vi "ToshibaComms.vi"(0 "FPGA VI Reference In":T8, 1 "PC Data In":T7, 3 "ES String Data Array In":T3, 4 "ES System Data In":T5={"Voltage"=0.0, "Current"=0.0, "SOC Avg"=0.0, "Faults"=0, "Alarms"=0, "Number of Strings"=0, "Max Temp"=0, "Min Temp"=0, "Max Cell Voltage"=0.0, "Min Cell Voltage"=0.0, "Energy Capacity (kWh)"=0.0, "Energy Remaining (kWh)"=0.0, "SOC Min"=0.0, "SOC Max"=0.0, "ES Fault"=FALSE, "String Selector"=enum."3 Strings"}, 5 "Error In":errorcluster, 6 "Contactor 2 Closed?":bool, 8 "Contactor 1 Closed?":bool) -> (10 "String A Com Fault":bool, 11 "Module Indicators 1":T1, 12 "String B Com Fault":bool, 14 "FPGA VI Reference Out":T8, 15 "Current Limit Parameters Out":T2, 17 "ES String Data Array Out":T3, 18 "ES System Data Out":T5={"Voltage"=0.0, "Current"=0.0, "SOC Avg"=0.0, "Faults"=0, "Alarms"=0, "Number of Strings"=0, "Max Temp"=0, "Min Temp"=0, "Max Cell Voltage"=0.0, "Min Cell Voltage"=0.0, "Energy Capacity (kWh)"=0.0, "Energy Remaining (kWh)"=0.0, "SOC Min"=0.0, "SOC Max"=0.0, "ES Fault"=FALSE, "String Selector"=enum."3 Strings"}, 19 "Error Out":errorcluster)   [LabVIEW 2013]
uses:
  bigboss/trunk/sw/cRIO/Controls/FPGAReference BigBoss.ctl
  eng/trunk/ni/cRIO Master Files/Controls/PowerConversionData.ctl
  eng/trunk/ni/cRIO Master Files/Controls/EnergyStorageSystemData.ctl
  eng/trunk/ni/cRIO Master Files/Controls/StringSelector.ctl
  eng/trunk/ni/cRIO Master Files/Controls/EnergyStorageStringDataArray.ctl
  eng/trunk/ni/cRIO Master Files/Controls/EnergyStorageStringData.ctl
  eng/trunk/ni/cRIO Master Files/Controls/CurrentLimitParameters.ctl
  <vilib>/rvi/interface/nirviMethod/nirviMethod.xnode
  Builds/FPGA Bitfiles/FPGA BIGBOSS.lvbitx
  <vilib>/rvi/errors/niLvFpgaMergeErrorWithErrorCode.vi
  <vilib>/FPGAPlugInAG/cRIO-9068/niLvFpga_ReadFifo_cRIO-9068.vi
  <vilib>/FPGAPlugInAG/cRIO-9068/niLvFpga_WriteFifo_cRIO-9068.vi
panel:
  out "Module Indicators 2":T1
  out "BMU heartbeat 2":bool
  out "BMU heartbeat 1":bool
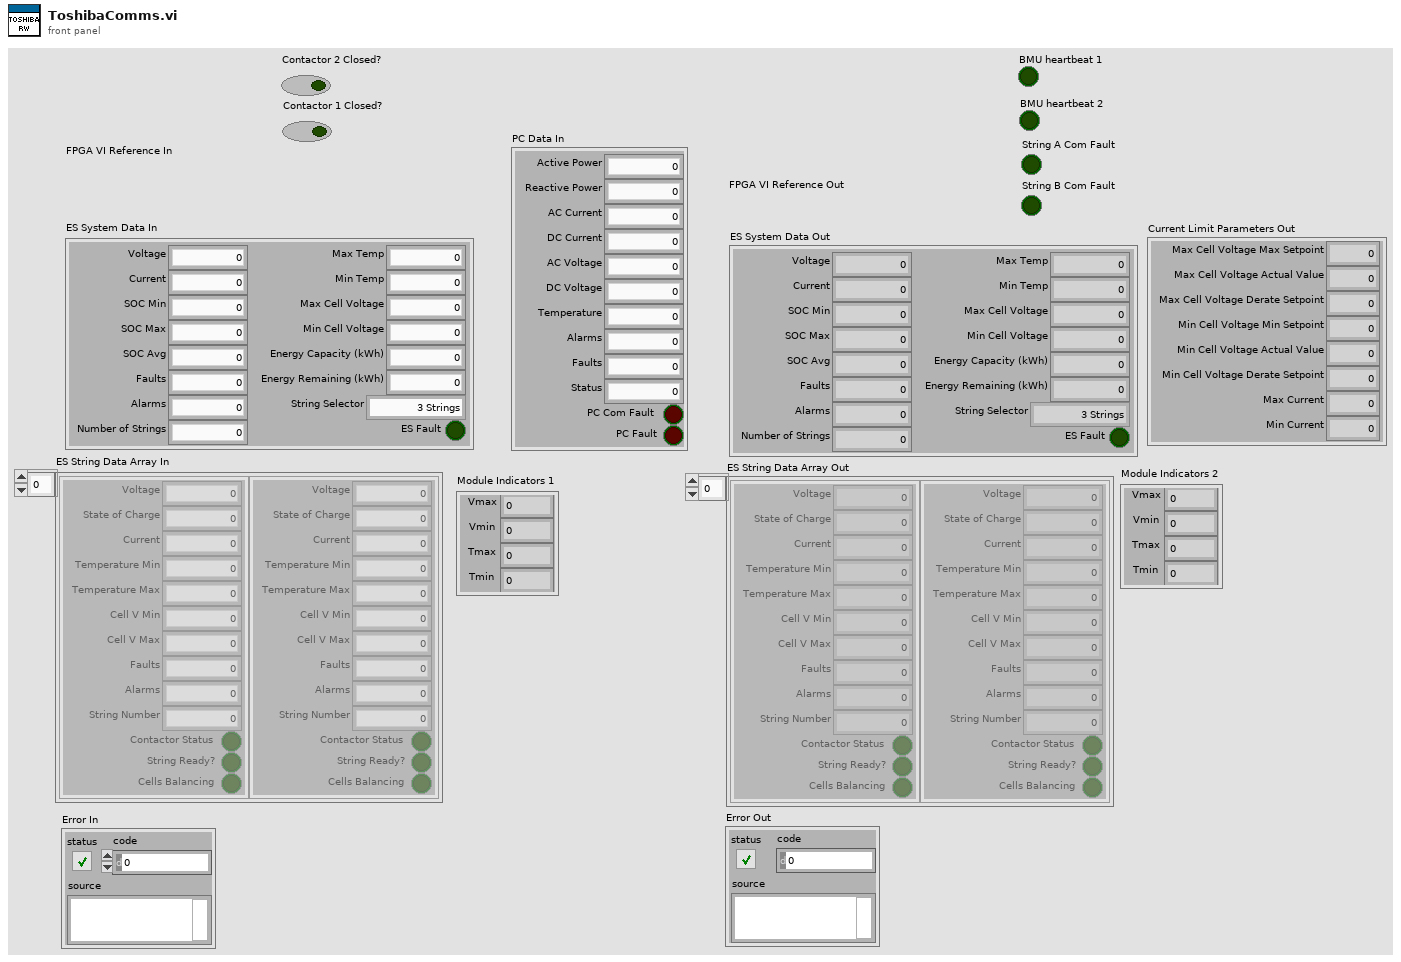
[diagram p1: front panel]
types:
  T1 = cluster{"Vmax":i16, "Vmin":i16, "Tmax":i16, "Tmin":i16}
  T2 = typedef "CurrentLimitParameters.ctl" = cluster{"Max Cell Voltage Max Setpoint":dbl, "Max Cell Voltage Actual Value":dbl, "Max Cell Voltage Derate Setpoint":dbl, "Min Cell Voltage Min Setpoint":dbl, "Min Cell Voltage Actual Value":dbl, "Min Cell Voltage Derate Setpoint":dbl, "Max Current":dbl, "Min Current":dbl}
  T3 = typedef "EnergyStorageStringDataArray.ctl" = T4[]
  T4 = typedef "EnergyStorageStringData.ctl" = cluster{"Voltage":sgl, "State of Charge":sgl, "Current":sgl, "Temperature Min":i16, "Temperature Max":i16, "Faults":u16, "Alarms":u16, "String Number":u16, "Contactor Status":bool, "String Ready?":bool, "Cells Balancing":bool, "Cell V Max":dbl, "Cell V Min":dbl}
  T5 = typedef "EnergyStorageSystemData.ctl" = cluster{"Voltage":sgl, "Current":sgl, "SOC Avg":sgl, "Faults":u16, "Alarms":u16, "Number of Strings":u16, "Max Temp":i16, "Min Temp":i16, "Max Cell Voltage":sgl, "Min Cell Voltage":sgl, "Energy Capacity (kWh)":sgl, "Energy Remaining (kWh)":sgl, "SOC Min":sgl, "SOC Max":sgl, "ES Fault":bool, "String Selector":T6}
  T6 = typedef "StringSelector.ctl" = enum16{"1 String (1)", "1 String (2)", "1 String (3)", "2 Strings (1, 2)", "2 Strings (2, 3)", "2 Strings (1, 3)", "3 Strings"}
  T7 = typedef "PowerConversionData.ctl" = cluster{"Active Power":sgl, "Reactive Power":sgl, "AC Current":sgl, "DC Current":sgl, "AC Voltage":sgl, "DC Voltage":sgl, "Temperature":sgl, "Alarms":u16, "Faults":u16, "Status":u16, "PC Fault":bool, "PC Com Fault":bool}
  T8 = typedef "FPGAReference BigBoss.ctl" = refnum<k20>
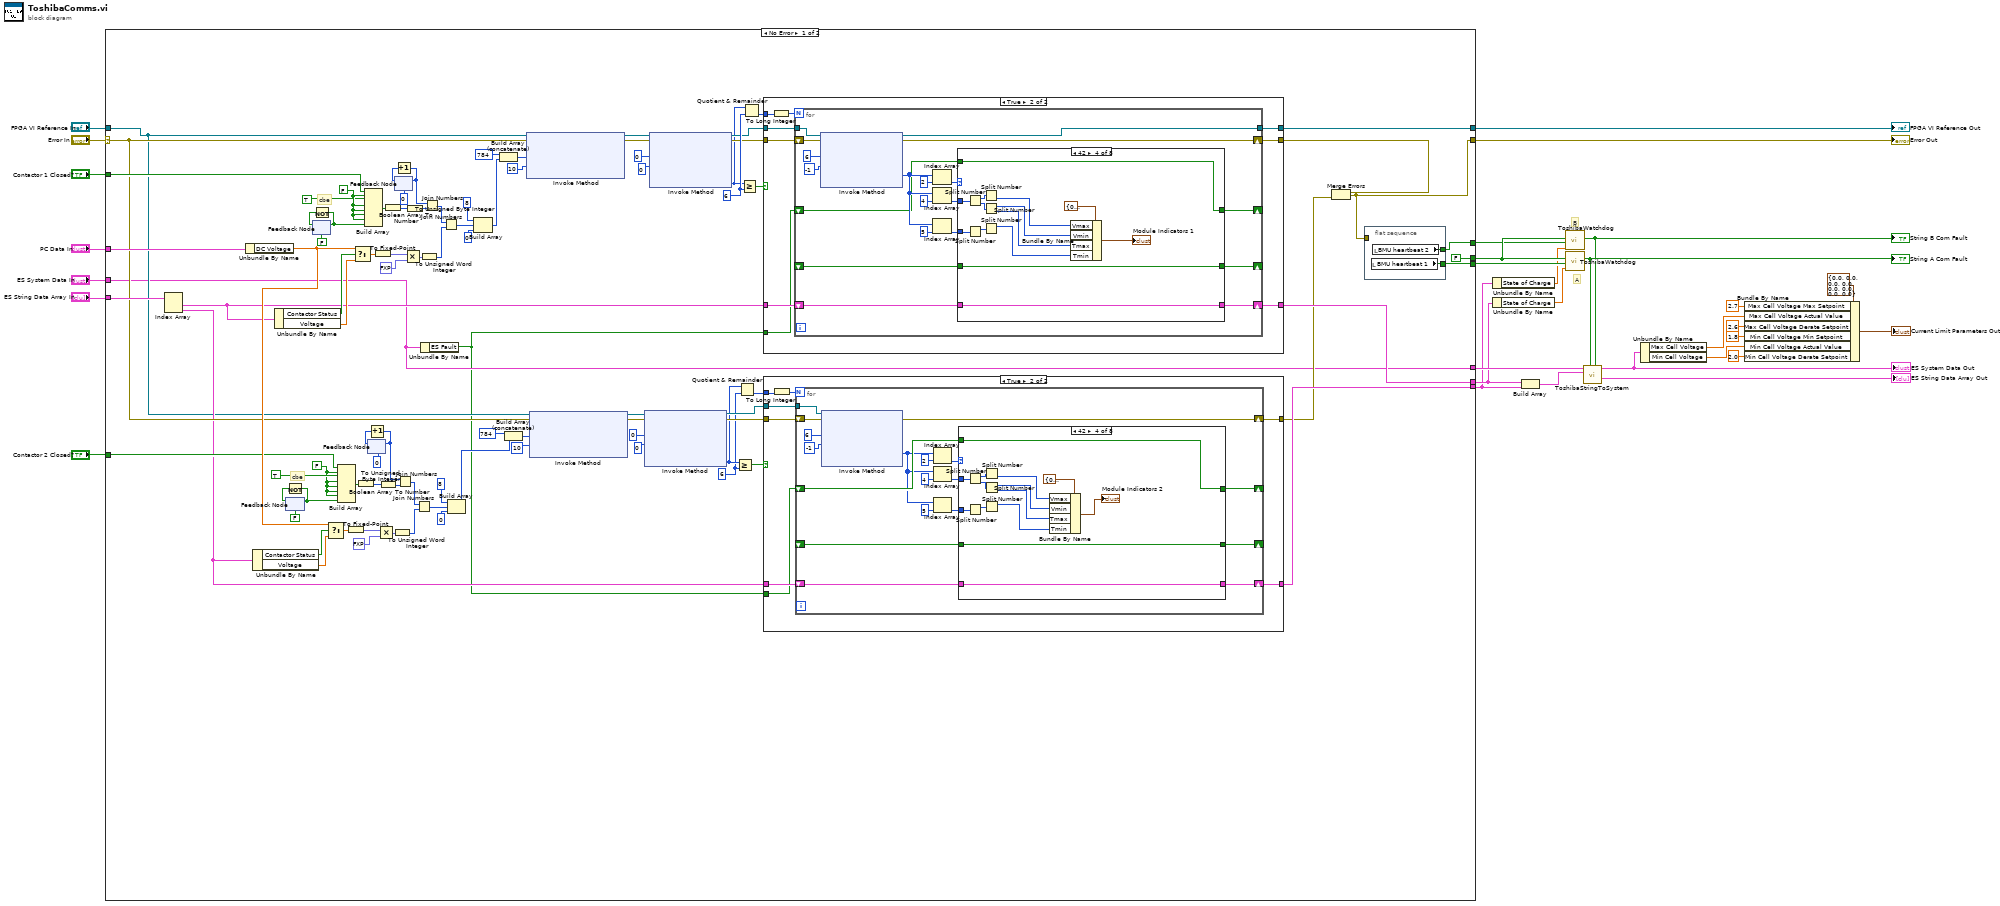
[diagram p0: block diagram]
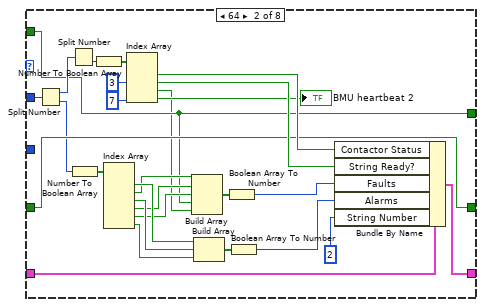
[diagram p4: hidden frame]
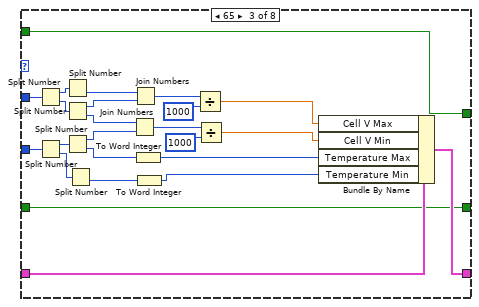
[diagram p5: hidden frame]
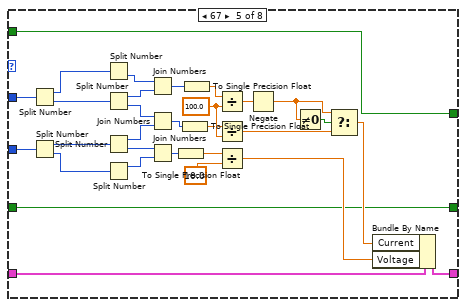
[diagram p6: hidden frame]
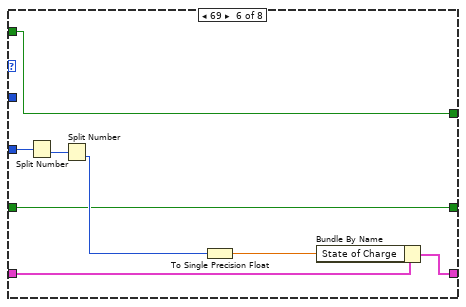
[diagram p7: hidden frame]
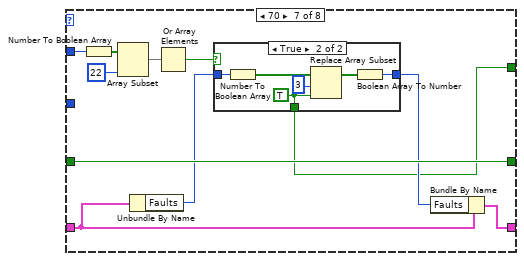
[diagram p8: hidden frame]
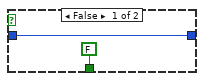
[diagram p9: hidden frame]
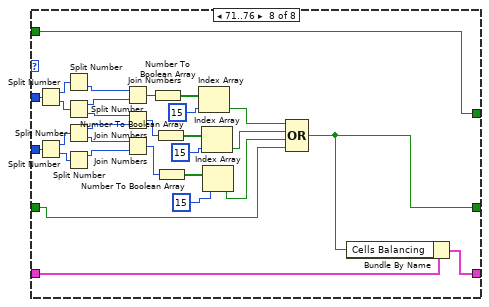
[diagram p10: hidden frame]
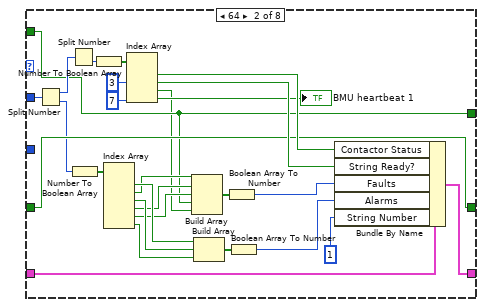
[diagram p13: hidden frame]
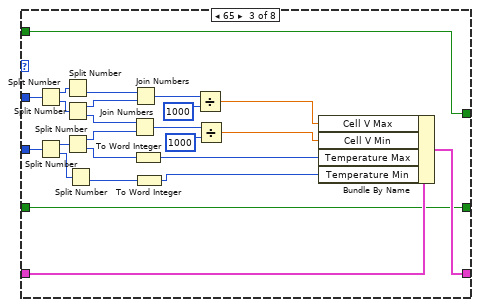
[diagram p14: hidden frame]
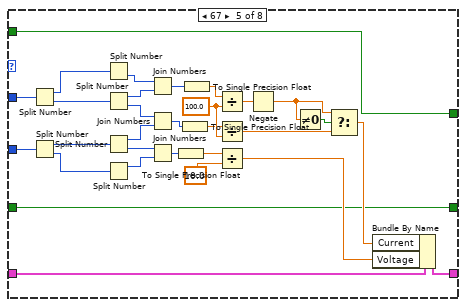
[diagram p15: hidden frame]
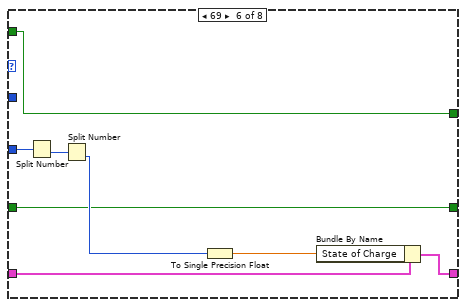
[diagram p16: hidden frame]
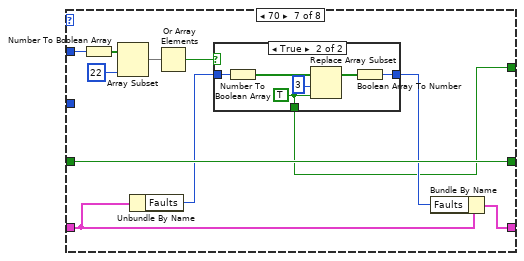
[diagram p17: hidden frame]
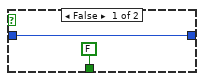
[diagram p18: hidden frame]
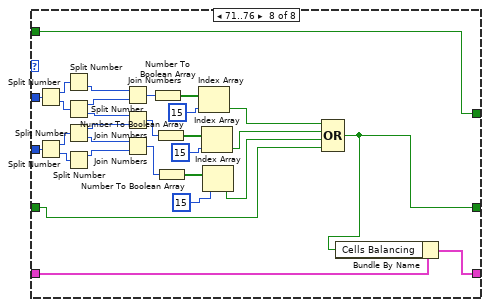
[diagram p19: hidden frame]
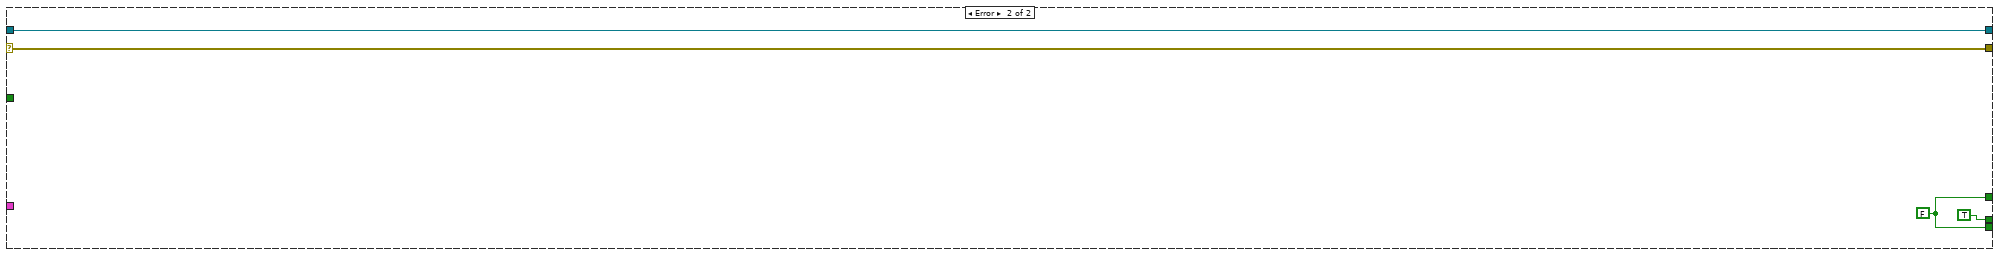
[diagram p20: hidden frame]
diagram:
  # "B"
  # "A"
  n1 = case shown="No Error" "Error In" {
    selector: "Error In" -> [w79 w495]
    tunnel: "FPGA VI Reference In" -> [w33 w494]
    tunnel: [w34 w494] -> w29
    tunnel: [w71 w495] -> w28
    tunnel: "PC Data In" -> [w122 _]
    tunnel: "Contactor 1 Closed?" -> [w121 _]
    tunnel: "ES System Data In" -> [w32 _]
    tunnel: [w32 _] -> w9
    tunnel: [FALSE TRUE] -> w12
    tunnel: "ES String Data Array In" -> [w82 _]
    tunnel: [w119 w492] -> w14
    tunnel: "Contactor 2 Closed?" -> [w86 _]
    tunnel: [w78 w492] -> w11
    tunnel: [w75 _] -> w6
    tunnel: [w74 _] -> w5
    frame No Error {
      w37 = u32 6 ("y")
      w49 = FALSE (".not. x?")
      w106 = FALSE (".not. x?")
      w118 = u32 6 ("y")
      # "cbe"
      # "cbe"
      n2 = Index Array(array=w82) -> (element #1=w77:T4, element #2=w76:T4)  [unwired: 2 in]
      n3 = Unbundle By Name(w122) -> ("DC Voltage"=w87:sgl)
      n4 = Unbundle By Name(w76) -> ("Contactor Status"=w45:bool, "Voltage"=w46:sgl)
      n5 = Unbundle By Name(w77) -> ("Contactor Status"=w84:bool, "Voltage"=w83:sgl)
      n6 = feedback #1(FALSE) -> (w60:bool)
      n7 = Not(x=w60) -> (.not. x?=w59:bool)
      n8 = feedback-in #1(w59) -> ()
      n9 = feedback #2(FALSE) -> (w95:bool)
      n10 = Not(x=w95) -> (.not. x?=w96:bool)
      n11 = feedback-in #2(w96) -> ()
      n12 = Select(t=w87, s=w45, f=w46) -> (s? t:f=w67:sgl)
      n13 = Build Array(w86, w49, TRUE ("Cell Balance 2"), w49, w49, w49, w49, w59) -> (w52:bool[])
      n14 = To Fixed-Point(number=w67) -> (fixed-point=w48:fxp<+,16,9>)  [unwired: 1 in]
      n15 = Select(t=w87, s=w84, f=w83) -> (s? t:f=w88:sgl)
      n16 = Boolean Array To Number(Boolean array=w52) -> (number=w51:u32)
      n17 = Build Array(w121, w106, TRUE, w106, w106, w106, w106, w96) -> (w103:bool[])
      n18 = feedback #3(u8 0) -> (w62:u8)
      n19 = Increment(x=w62) -> (x+1=w63:u8)
      n20 = feedback-in #3(w63) -> ()
      n21 = To Fixed-Point(number=w88) -> (fixed-point=w107:fxp<+,16,9>)  [unwired: 1 in]
      n22 = Multiply(x=w48, y=fxp<+,16,9> 10.0) -> (x*y=w54:fxp<+,16,16>)
      n23 = To Unsigned Byte Integer(number=w51) -> (unsigned 8bit integer=w50:u8)
      n24 = Boolean Array To Number(Boolean array=w103) -> (number=w104:u32)
      n25 = To Unsigned Word Integer(number=w54) -> (unsigned 16bit integer=w53:u16)
      n26 = feedback #4(u8 0) -> (w92:u8)
      n27 = Increment(x=w92) -> (x+1=w91:u8)
      n28 = feedback-in #4(w91) -> ()
      n29 = Join Numbers(hi=w63, lo=w50) -> ((hi.lo)=w56:u16)
      n30 = Multiply(x=w107, y=fxp<+,16,9> 10.0) -> (x*y=w101:fxp<+,16,16>)
      n31 = To Unsigned Byte Integer(number=w104) -> (unsigned 8bit integer=w105:u8)
      n32 = Join Numbers(hi=w56, lo=w53) -> ((hi.lo)=w66:u32)
      n33 = To Unsigned Word Integer(number=w101) -> (unsigned 16bit integer=w102:u16)
      n34 = Unbundle By Name(w32) -> ("ES Fault"=w31:bool)
      n35 = Join Numbers(hi=w91, lo=w105) -> ((hi.lo)=w99:u16)
      n36 = Join Numbers(hi=w99, lo=w102) -> ((hi.lo)=w89:u32)
      n37 = Build Array(u32 8, w66, u32 0 ("CAN Word 2")) -> (w47:u32[])
      n38 = Build Array(u32 8, w89, u32 0 ("CAN Word 2")) -> (w94:u32[])
      n39 = Build Array (concatenate)(u32 784, w94) -> (w109:u32[])
      n40 = Build Array (concatenate)(u32 784, w47) -> (w69:u32[])
      n41 = xnode "Invoke Method"("FPGA VI Reference In"=w33, "error in"=w79, "Data"=w109, "Timeout (ms)"=10) -> ("FPGA VI Reference Out"=w81:T8, "error out"=w80:errorcluster)  [unwired: 1 out]
      n42 = xnode "Invoke Method"("FPGA VI Reference In"=w33, "error in"=w79, "Data"=w69, "Timeout (ms)"=10) -> ("FPGA VI Reference Out"=w42:T8, "error out"=w41:errorcluster)  [unwired: 1 out]
      n43 = xnode "Invoke Method"("FPGA VI Reference In"=w42, "error in"=w41, "Number of Elements"=u32 0, "Timeout (ms)"=0) -> ("FPGA VI Reference Out"=w39:T8, "error out"=w40:errorcluster, "Elements Remaining"=w38:u32)  [unwired: 1 out]
      n44 = xnode "Invoke Method"("FPGA VI Reference In"=w81, "error in"=w80, "Number of Elements"=u32 0, "Timeout (ms)"=0) -> ("FPGA VI Reference Out"=w114:T8, "error out"=w115:errorcluster, "Elements Remaining"=w111:u32)  [unwired: 1 out]
      n45 = Greater Or Equal?(x=w38, y=w37) -> (x >= y?=w35:bool)
      n46 = Quotient & Remainder(x=w38, y=w37) -> (floor(x/y)=w36:u32)  [unwired: 1 out]
      n47 = Greater Or Equal?(x=w111, y=w118) -> (x >= y?=w113:bool)
      n48 = Quotient & Remainder(x=w111, y=w118) -> (floor(x/y)=w112:u32)  [unwired: 1 out]
      n49 = case shown="True" w113 {
        tunnel: w115 -> [w308 w318]
        tunnel: w114 -> [w309 w317]
        tunnel: w112 -> [_ w316]
        tunnel: [w308 w314] -> w72
        tunnel: [w309 w313] -> w34
        tunnel: [w307 w311] -> w75
        tunnel: w77 -> [w307 w312]
        tunnel: w31 -> [_ w310]
        frame False {
        }
        frame True {
          n50 = To Long Integer(number=w316) -> (32bit integer=w315:i32)
          n51 = for {
            N: w315 -> [_]
            tunnel: w317 -> [w337]
            tunnel: [w334] -> w313
            shift-right: [w332] -> w314
            shift-left: w318 -> [w333]
            shift-right: [w320] -> w311
            shift-left: w312 -> [w321]
            shift-right: [w325] -> _
            shift-left: _ -> [w324]
            shift-right: [w323] -> _
            shift-left: w310 -> [w322]
            n52 = xnode "Invoke Method"("FPGA VI Reference In"=w337, "error in"=w333, "Number of Elements"=u32 6, "Timeout (ms)"=-1) -> ("FPGA VI Reference Out"=w334:T8, "error out"=w332:errorcluster, "Data"=w326:u32[])  [unwired: 1 out]
            n53 = Index Array(array=w326, index=2) -> (element=w319:u32)
            n54 = Index Array(array=w326, index=4) -> (element=w330:u32)
            n55 = Index Array(array=w326, index=5) -> (element=w331:u32)
            n56 = case shown="42" w319 {
              tunnel: w330 -> [_ w364 w391 w405 w435 _ w450 w491]
              tunnel: w331 -> [_ _ w387 w401 w431 w443 _ w490]
              tunnel: w321 -> [w340 w357 w377 w398 w415 w439 w444 w467]
              tunnel: [w340 w358 w376 w398 w414 w438 w449 w466] -> w320
              tunnel: [w339 w356 w375 w399 w413 w437 w454 w464] -> w325
              tunnel: w324 -> [w339 w356 w375 w399 w413 w437 w454 w465]
              tunnel: [w338 w342 w370 w400 w406 w436 w445 w463] -> w323
              tunnel: w322 -> [w338 w342 w370 w400 w406 w436 _ w463]
              frame 0, Default {
              }
              frame 64 {
                n57 = Split Number(x=w364) -> (hi(x)=w366:u16, lo(x)=w354:u16)
                n58 = Split Number(x=w366) -> (lo(x)=w365:u8)  [unwired: 1 out]
                n59 = Number To Boolean Array(number=w354) -> (Boolean array=w353:bool[])
                n60 = Number To Boolean Array(number=w365) -> (Boolean array=w367:bool[])
                n61 = Index Array(array=w353) -> (element #1=w352:bool, element #2=w348:bool, element #3=w351:bool, element #4=w347:bool, element #5=w346:bool, element #6=w350:bool)  [unwired: 6 in]
                n62 = Index Array(array=w367, index #2=3 ("index"), index #4=7 ("index")) -> (element #1=w363:bool, element #2=w361:bool, element #3=w341:bool, element #4=→"BMU heartbeat 1":bool)  [unwired: 2 in]
                n63 = Build Array(w348, w347, w346, w342, w341) -> (w345:bool[])
                n64 = Build Array(w352, w351, w350) -> (w349:bool[])
                n65 = Boolean Array To Number(Boolean array=w345) -> (number=w344:u32)
                n66 = Boolean Array To Number(Boolean array=w349) -> (number=w343:u32)
                n67 = Bundle By Name(cluster=w357, "Contactor Status"=w363, "String Ready?"=w361, "Faults"=w344, "Alarms"=w343, "String Number"=u16 1) -> (w358:T4)
              }
              frame 65 {
                n68 = Split Number(x=w391) -> (hi(x)=w390:u16, lo(x)=w389:u16)
                n69 = Split Number(x=w387) -> (hi(x)=w388:u16, lo(x)=w373:u16)
                n70 = Split Number(x=w390) -> (lo(x)=w386:u8)  [unwired: 1 out]
                n71 = Split Number(x=w389) -> (hi(x)=w385:u8, lo(x)=w384:u8)
                n72 = Split Number(x=w388) -> (hi(x)=w383:u8, lo(x)=w378:u8)
                n73 = Split Number(x=w373) -> (lo(x)=w372:u8)  [unwired: 1 out]
                n74 = Join Numbers(hi=w384, lo=w383) -> ((hi.lo)=w379:u16)
                n75 = Join Numbers(hi=w386, lo=w385) -> ((hi.lo)=w382:u16)
                n76 = To Word Integer(number=w378) -> (16bit integer=w374:i16)
                n77 = To Word Integer(number=w372) -> (16bit integer=w371:i16)
                n78 = Divide(x=w382, y=u16 1000) -> (x/y=w369:dbl)
                n79 = Divide(x=w379, y=u16 1000) -> (x/y=w368:dbl)
                n80 = Bundle By Name(cluster=w377, "Cell V Max"=w369, "Cell V Min"=w368, "Temperature Max"=w374, "Temperature Min"=w371) -> (w376:T4)
              }
              frame 66 {
                n81 = Split Number(x=w405) -> (hi(x)=w404:u16, lo(x)=w403:u16)
                n82 = Split Number(x=w401) -> (hi(x)=w402:u16)  [unwired: 1 out]
                n83 = Split Number(x=w404) -> (lo(x)=w395:u8)  [unwired: 1 out]
                n84 = Split Number(x=w403) -> (hi(x)=w394:u8, lo(x)=w393:u8)
                n85 = Split Number(x=w402) -> (hi(x)=w392:u8)  [unwired: 1 out]
                n86 = Bundle By Name(cluster=T1 {"Vmax"=0, "Vmin"=0, "Tmax"=0, "Tmin"=0} ("Module Indicators"), "Vmax"=w395, "Vmin"=w394, "Tmax"=w393, "Tmin"=w392) -> (→"Module Indicators 1":T1)
              }
              frame 67 {
                w411 = sgl 100.0 ("y")
                n87 = Split Number(x=w435) -> (hi(x)=w434:u16, lo(x)=w433:u16)
                n88 = Split Number(x=w431) -> (hi(x)=w432:u16, lo(x)=w420:u16)
                n89 = Split Number(x=w434) -> (lo(x)=w430:u8)  [unwired: 1 out]
                n90 = Split Number(x=w433) -> (hi(x)=w429:u8, lo(x)=w428:u8)
                n91 = Split Number(x=w432) -> (hi(x)=w427:u8, lo(x)=w424:u8)
                n92 = Split Number(x=w420) -> (hi(x)=w421:u8)  [unwired: 1 out]
                n93 = Join Numbers(hi=w430, lo=w429) -> ((hi.lo)=w426:u16)
                n94 = Join Numbers(hi=w428, lo=w427) -> ((hi.lo)=w425:u16)
                n95 = Join Numbers(hi=w424, lo=w421) -> ((hi.lo)=w423:u16)
                n96 = To Single Precision Float(number=w423) -> (single precision float=w409:sgl)
                n97 = To Single Precision Float(number=w425) -> (single precision float=w410:sgl)
                n98 = To Single Precision Float(number=w426) -> (single precision float=w412:sgl)
                n99 = Divide(x=w412, y=w411) -> (x/y=w418:sgl)
                n100 = Divide(x=w410, y=w411) -> (x/y=w407:sgl)
                n101 = Divide(x=w409, y=sgl 10.0) -> (x/y=w416:sgl)
                n102 = Negate(x=w418) -> (-x=w408:sgl)
                n103 = Not Equal To 0?(x=w408) -> (x != 0?=w419:bool)
                n104 = Select(t=w408, s=w419, f=w407) -> (s? t:f=w417:sgl)
                n105 = Bundle By Name(cluster=w415, "Current"=w417, "Voltage"=w416) -> (w414:T4)
              }
              frame 69 {
                n106 = Split Number(x=w443) -> (lo(x)=w442:u16)  [unwired: 1 out]
                n107 = Split Number(x=w442) -> (lo(x)=w440:u8)  [unwired: 1 out]
                n108 = To Single Precision Float(number=w440) -> (single precision float=w441:sgl)
                n109 = Bundle By Name(cluster=w439, "State of Charge"=w441) -> (w438:T4)
              }
              frame 70 {
                n110 = Number To Boolean Array(number=w450) -> (Boolean array=w453:bool[])
                n111 = Array Subset(array=w453, length=22) -> (w451:bool[])  [unwired: 1 in]
                n112 = Unbundle By Name(w444) -> ("Faults"=w448:u16)
                n113 = Or Array Elements(Boolean array=w451) -> (logical OR=w447:bool)
                n114 = case shown="True" w447 {
                  tunnel: w448 -> [w456 w462]
                  tunnel: [w456 w458] -> w446
                  tunnel: [FALSE ("new element/subarray") w457] -> w445
                  frame False {
                  }
                  frame True {
                    w457 = TRUE ("new element/subarray")
                    n115 = Number To Boolean Array(number=w462) -> (Boolean array=w461:bool[])
                    n116 = Replace Array Subset(array=w461, new element=w457, index=3) -> (w459:bool[])
                    n117 = Boolean Array To Number(Boolean array=w459) -> (number=w458:u32)
                  }
                }
                n118 = Bundle By Name(cluster=w444, "Faults"=w446) -> (w449:T4)
              }
              frame 71..76 {
                n119 = Split Number(x=w491) -> (hi(x)=w489:u16, lo(x)=w488:u16)
                n120 = Split Number(x=w490) -> (hi(x)=w487:u16, lo(x)=w486:u16)
                n121 = Split Number(x=w489) -> (lo(x)=w485:u8)  [unwired: 1 out]
                n122 = Split Number(x=w488) -> (hi(x)=w484:u8, lo(x)=w483:u8)
                n123 = Split Number(x=w487) -> (hi(x)=w482:u8, lo(x)=w481:u8)
                n124 = Split Number(x=w486) -> (hi(x)=w480:u8)  [unwired: 1 out]
                n125 = Join Numbers(hi=w485, lo=w484) -> ((hi.lo)=w479:u16)
                n126 = Join Numbers(hi=w483, lo=w482) -> ((hi.lo)=w473:u16)
                n127 = Join Numbers(hi=w481, lo=w480) -> ((hi.lo)=w469:u16)
                n128 = Number To Boolean Array(number=w479) -> (Boolean array=w478:bool[])
                n129 = Number To Boolean Array(number=w473) -> (Boolean array=w475:bool[])
                n130 = Number To Boolean Array(number=w469) -> (Boolean array=w471:bool[])
                n131 = Index Array(array=w478, index=15) -> (element=w476:bool)
                n132 = Index Array(array=w475, index=15) -> (element=w472:bool)
                n133 = Index Array(array=w471, index=15) -> (element=w468:bool)
                n134 = Compound Arithmetic op=OR(w476, w472, w468, w465) -> (w464:bool)
                n135 = Bundle By Name(cluster=w467, "Cells Balancing"=w464) -> (w466:T4)
              }
            }
          }
        }
      }
      n136 = case shown="True" w35 {
        tunnel: w40 -> [w124 w132]
        tunnel: w39 -> [_ w131]
        tunnel: w36 -> [_ w130]
        tunnel: [w124 w128] -> w73
        tunnel: [w123 w126] -> w74
        tunnel: w76 -> [w123 w127]
        tunnel: w31 -> [_ w125]
        frame False {
        }
        frame True {
          n137 = To Long Integer(number=w130) -> (32bit integer=w129:i32)
          n138 = for {
            N: w129 -> [_]
            tunnel: w131 -> [w135]
            shift-right: [w147] -> w128
            shift-left: w132 -> [w148]
            shift-right: [w136] -> w126
            shift-left: w127 -> [w137]
            shift-right: [w141] -> _
            shift-left: _ -> [w140]
            shift-right: [w139] -> _
            shift-left: w125 -> [w138]
            n139 = xnode "Invoke Method"("FPGA VI Reference In"=w135, "error in"=w148, "Number of Elements"=u32 6, "Timeout (ms)"=-1) -> ("error out"=w147:errorcluster, "Data"=w134:u32[])  [unwired: 2 out]
            n140 = Index Array(array=w134, index=2) -> (element=w133:u32)
            n141 = Index Array(array=w134, index=4) -> (element=w145:u32)
            n142 = Index Array(array=w134, index=5) -> (element=w146:u32)
            n143 = case shown="42" w133 {
              tunnel: w145 -> [_ w177 w204 w218 w248 _ w263 w304]
              tunnel: w146 -> [_ _ w200 w214 w244 w256 _ w303]
              tunnel: w137 -> [w153 w170 w190 w212 w228 w252 w257 w280]
              tunnel: [w153 w171 w189 w212 w227 w251 w262 w279] -> w136
              tunnel: [w152 w169 w188 w211 w226 w250 w267 w277] -> w141
              tunnel: w140 -> [w152 w169 w188 w211 w226 w250 w267 w278]
              tunnel: [w151 w155 w183 w213 w219 w249 w258 w276] -> w139
              tunnel: w138 -> [w151 w155 w183 w213 w219 w249 _ w276]
              frame 0, Default {
              }
              frame 64 {
                n144 = Split Number(x=w177) -> (hi(x)=w179:u16, lo(x)=w167:u16)
                n145 = Split Number(x=w179) -> (lo(x)=w178:u8)  [unwired: 1 out]
                n146 = Number To Boolean Array(number=w167) -> (Boolean array=w166:bool[])
                n147 = Number To Boolean Array(number=w178) -> (Boolean array=w180:bool[])
                n148 = Index Array(array=w166) -> (element #1=w165:bool, element #2=w161:bool, element #3=w164:bool, element #4=w160:bool, element #5=w159:bool, element #6=w163:bool)  [unwired: 6 in]
                n149 = Index Array(array=w180, index #2=3 ("index"), index #4=7 ("index")) -> (element #1=w176:bool, element #2=w174:bool, element #3=w154:bool, element #4=→"BMU heartbeat 2":bool)  [unwired: 2 in]
                n150 = Build Array(w161, w160, w159, w155, w154) -> (w158:bool[])
                n151 = Build Array(w165, w164, w163) -> (w162:bool[])
                n152 = Boolean Array To Number(Boolean array=w158) -> (number=w157:u32)
                n153 = Boolean Array To Number(Boolean array=w162) -> (number=w156:u32)
                n154 = Bundle By Name(cluster=w170, "Contactor Status"=w176, "String Ready?"=w174, "Faults"=w157, "Alarms"=w156, "String Number"=u16 2) -> (w171:T4)
              }
              frame 65 {
                n155 = Split Number(x=w204) -> (hi(x)=w203:u16, lo(x)=w202:u16)
                n156 = Split Number(x=w200) -> (hi(x)=w201:u16, lo(x)=w186:u16)
                n157 = Split Number(x=w203) -> (lo(x)=w199:u8)  [unwired: 1 out]
                n158 = Split Number(x=w202) -> (hi(x)=w198:u8, lo(x)=w197:u8)
                n159 = Split Number(x=w201) -> (hi(x)=w196:u8, lo(x)=w191:u8)
                n160 = Split Number(x=w186) -> (lo(x)=w185:u8)  [unwired: 1 out]
                n161 = Join Numbers(hi=w197, lo=w196) -> ((hi.lo)=w192:u16)
                n162 = Join Numbers(hi=w199, lo=w198) -> ((hi.lo)=w195:u16)
                n163 = To Word Integer(number=w191) -> (16bit integer=w187:i16)
                n164 = To Word Integer(number=w185) -> (16bit integer=w184:i16)
                n165 = Divide(x=w195, y=u16 1000) -> (x/y=w182:dbl)
                n166 = Divide(x=w192, y=u16 1000) -> (x/y=w181:dbl)
                n167 = Bundle By Name(cluster=w190, "Cell V Max"=w182, "Cell V Min"=w181, "Temperature Max"=w187, "Temperature Min"=w184) -> (w189:T4)
              }
              frame 66 {
                n168 = Split Number(x=w218) -> (hi(x)=w217:u16, lo(x)=w216:u16)
                n169 = Split Number(x=w214) -> (hi(x)=w215:u16)  [unwired: 1 out]
                n170 = Split Number(x=w217) -> (lo(x)=w208:u8)  [unwired: 1 out]
                n171 = Split Number(x=w216) -> (hi(x)=w207:u8, lo(x)=w206:u8)
                n172 = Split Number(x=w215) -> (hi(x)=w205:u8)  [unwired: 1 out]
                n173 = Bundle By Name(cluster=T1 {"Vmax"=0, "Vmin"=0, "Tmax"=0, "Tmin"=0} ("Module Indicators"), "Vmax"=w208, "Vmin"=w207, "Tmax"=w206, "Tmin"=w205) -> (→"Module Indicators 2":T1)
              }
              frame 67 {
                w224 = sgl 100.0 ("y")
                n174 = Split Number(x=w248) -> (hi(x)=w247:u16, lo(x)=w246:u16)
                n175 = Split Number(x=w244) -> (hi(x)=w245:u16, lo(x)=w233:u16)
                n176 = Split Number(x=w247) -> (lo(x)=w243:u8)  [unwired: 1 out]
                n177 = Split Number(x=w246) -> (hi(x)=w242:u8, lo(x)=w241:u8)
                n178 = Split Number(x=w245) -> (hi(x)=w240:u8, lo(x)=w237:u8)
                n179 = Split Number(x=w233) -> (hi(x)=w234:u8)  [unwired: 1 out]
                n180 = Join Numbers(hi=w243, lo=w242) -> ((hi.lo)=w239:u16)
                n181 = Join Numbers(hi=w241, lo=w240) -> ((hi.lo)=w238:u16)
                n182 = Join Numbers(hi=w237, lo=w234) -> ((hi.lo)=w236:u16)
                n183 = To Single Precision Float(number=w236) -> (single precision float=w222:sgl)
                n184 = To Single Precision Float(number=w238) -> (single precision float=w223:sgl)
                n185 = To Single Precision Float(number=w239) -> (single precision float=w225:sgl)
                n186 = Divide(x=w225, y=w224) -> (x/y=w231:sgl)
                n187 = Divide(x=w223, y=w224) -> (x/y=w220:sgl)
                n188 = Divide(x=w222, y=sgl 10.0) -> (x/y=w229:sgl)
                n189 = Negate(x=w231) -> (-x=w221:sgl)
                n190 = Not Equal To 0?(x=w221) -> (x != 0?=w232:bool)
                n191 = Select(t=w221, s=w232, f=w220) -> (s? t:f=w230:sgl)
                n192 = Bundle By Name(cluster=w228, "Current"=w230, "Voltage"=w229) -> (w227:T4)
              }
              frame 69 {
                n193 = Split Number(x=w256) -> (lo(x)=w255:u16)  [unwired: 1 out]
                n194 = Split Number(x=w255) -> (lo(x)=w253:u8)  [unwired: 1 out]
                n195 = To Single Precision Float(number=w253) -> (single precision float=w254:sgl)
                n196 = Bundle By Name(cluster=w252, "State of Charge"=w254) -> (w251:T4)
              }
              frame 70 {
                n197 = Number To Boolean Array(number=w263) -> (Boolean array=w266:bool[])
                n198 = Array Subset(array=w266, length=22) -> (w264:bool[])  [unwired: 1 in]
                n199 = Unbundle By Name(w257) -> ("Faults"=w261:u16)
                n200 = Or Array Elements(Boolean array=w264) -> (logical OR=w260:bool)
                n201 = case shown="True" w260 {
                  tunnel: w261 -> [w269 w275]
                  tunnel: [w269 w271] -> w259
                  tunnel: [FALSE ("new element/subarray") w270] -> w258
                  frame False {
                  }
                  frame True {
                    w270 = TRUE ("new element/subarray")
                    n202 = Number To Boolean Array(number=w275) -> (Boolean array=w274:bool[])
                    n203 = Replace Array Subset(array=w274, new element=w270, index=3) -> (w272:bool[])
                    n204 = Boolean Array To Number(Boolean array=w272) -> (number=w271:u32)
                  }
                }
                n205 = Bundle By Name(cluster=w257, "Faults"=w259) -> (w262:T4)
              }
              frame 71..76 {
                n206 = Split Number(x=w304) -> (hi(x)=w302:u16, lo(x)=w301:u16)
                n207 = Split Number(x=w303) -> (hi(x)=w300:u16, lo(x)=w299:u16)
                n208 = Split Number(x=w302) -> (lo(x)=w298:u8)  [unwired: 1 out]
                n209 = Split Number(x=w301) -> (hi(x)=w297:u8, lo(x)=w296:u8)
                n210 = Split Number(x=w300) -> (hi(x)=w295:u8, lo(x)=w294:u8)
                n211 = Split Number(x=w299) -> (hi(x)=w293:u8)  [unwired: 1 out]
                n212 = Join Numbers(hi=w298, lo=w297) -> ((hi.lo)=w292:u16)
                n213 = Join Numbers(hi=w296, lo=w295) -> ((hi.lo)=w286:u16)
                n214 = Join Numbers(hi=w294, lo=w293) -> ((hi.lo)=w282:u16)
                n215 = Number To Boolean Array(number=w292) -> (Boolean array=w291:bool[])
                n216 = Number To Boolean Array(number=w286) -> (Boolean array=w288:bool[])
                n217 = Number To Boolean Array(number=w282) -> (Boolean array=w284:bool[])
                n218 = Index Array(array=w291, index=15) -> (element=w289:bool)
                n219 = Index Array(array=w288, index=15) -> (element=w285:bool)
                n220 = Index Array(array=w284, index=15) -> (element=w281:bool)
                n221 = Compound Arithmetic op=OR(w289, w285, w281, w278) -> (w277:bool)
                n222 = Bundle By Name(cluster=w280, "Cells Balancing"=w277) -> (w279:T4)
              }
            }
          }
        }
      }
      n223 = Merge Errors(w72, w73) -> (w71:errorcluster)
      n224 = flat-sequence {
        tunnel: [w306] -> w119
        tunnel: [w305] -> w78
        tunnel: w71 -> [_]
        frame #0 {
          n225 = local read "BMU heartbeat 1"() -> (w306:bool)
          n226 = local read "BMU heartbeat 2"() -> (w305:bool)
        }
      }
    }
    frame Error {
      w492 = FALSE ("BMU heartbeat")
    }
  }
  "FPGA VI Reference Out" <- w29
  "Error Out" <- w28
  n227 = Unbundle By Name(w5) -> ("State of Charge"=w2:sgl)
  n228 = Unbundle By Name(w6) -> ("State of Charge"=w1:sgl)
  n229 = Build Array(w6, w5) -> (w10:T4[])
  n230 = call "ToshibaWatchdog.vi"("State of Charge"=w2, "Heartbeat In"=w11, "ES Com Fault In"=w12) -> ("ES Com Fault Out"=w3:bool)  [unwired: 6 in]
  "String B Com Fault" <- w3
  n231 = call "ToshibaWatchdog.vi"("State of Charge"=w1, "Heartbeat In"=w14, "ES Com Fault In"=w12) -> ("ES Com Fault Out"=w4:bool)  [unwired: 6 in]
  "String A Com Fault" <- w4
  n232 = call "ToshibaStringToSystem.vi"("String B Com Fault"=w3, "String A Com Fault"=w4, "ES String Data Array In"=w10, "ES System Data In"=w9) -> ("ES String Data Array Out"=→"ES String Data Array Out":T3, "ES System Data Out"=w8:T5)  [unwired: 6 in]
  "ES System Data Out" <- w8
  n233 = Unbundle By Name(w8) -> ("Max Cell Voltage"=w16:sgl, "Min Cell Voltage"=w15:sgl)
  n234 = Bundle By Name(cluster=T2 {"Max Cell Voltage Max Setpoint"=0.0, "Max Cell Voltage Actual Value"=0.0, "Max Cell Voltage Derate Setpoint"=0.0, "Min Cell Voltage Min Setpoint"=0.0, "Min Cell Voltage Actual Value"=0.0, "Min Cell Voltage Derate Setpoint"=0.0, "Max Current"=0.0, "Min Current"=0.0} ("Current Limit Parameters Out"), "Max Cell Voltage Max Setpoint"=2.7, "Max Cell Voltage Actual Value"=w16, "Max Cell Voltage Derate Setpoint"=2.6, "Min Cell Voltage Min Setpoint"=1.8, "Min Cell Voltage Actual Value"=w15, "Min Cell Voltage Derate Setpoint"=2.0) -> (→"Current Limit Parameters Out":T2)
